vi "url_to_filename.vi"(8 "error in (no error)":errorcluster, 11 "url":string) -> (0 "error out":errorcluster, 3 "filename":path)   [LabVIEW 2015, in "lv-bin-wget.lvlib" / "v1.lvlib"]
uses:
  v1.lvlib
  <userlib>/antonio-alexander/lv-bin/lv-bin/public/api/v1/v1.lvlib
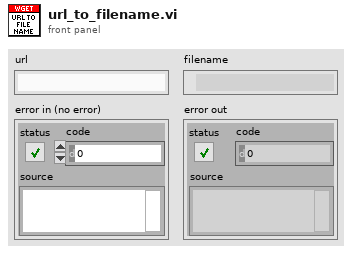
[diagram p1: front panel]
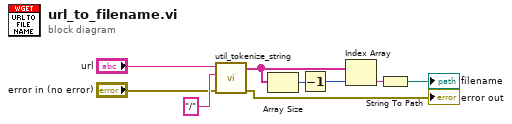
[diagram p0: block diagram]
diagram:
  n1 = call <userlib>:"util_tokenize_string.vi"("error in (no error)"="error in (no error)", "delimiter"="/", "input_string"="url") -> ("error out"=→"error out":errorcluster, "before_match []"=w5:string[])  [unwired: 6 in, 1 out]
  n2 = Array Size(array=w5) -> (size(s)=w4:i32)
  n3 = Decrement(x=w4) -> (x-1=w3:i32)
  n4 = Index Array(array=w5, index=w3) -> (element=w2:string)
  n5 = String To Path(string=w2) -> (path=→"filename":path)
